vi "readRestek.vi"(10 "Port Name":refnum<visa-resource-name>) -> (2 "lpm":dbl)   [LabVIEW 2020]
panel:
  out "element":string
  out "string array":string[](array[string])
  out "Read":string="This is simulation mode"
  # "Reads data stream from Restek ProFLOW 6000 volumetric flowmeter"
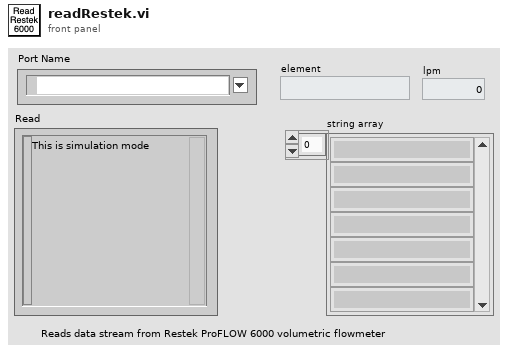
[diagram p1: front panel]
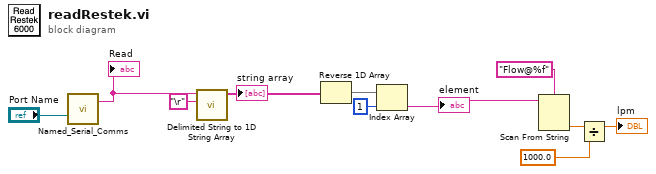
[diagram p0: block diagram]
diagram:
  n1 = call "Named_Serial_Comms.vi"("Port Name"="Port Name") -> ("Read"=w10:string)  [unwired: 10 in, 4 out]
  "Read" <- w10
  n2 = call <vilib>:"Delimited String to 1D String Array.vi"("delimiter"="\r", "delimited string"=w10) -> ("string array"=w8:string[])  [unwired: 9 in]
  "string array" <- w8
  n3 = Reverse 1D Array(array=w8) -> (reversed array=w7:string[])
  n4 = Index Array(array=w7, index=1) -> (element=w5:string)
  "element" <- w5
  n5 = Scan From String(format string="Flow@%f", input string=w5) -> (output 1=w4:dbl)  [unwired: 3 in, 3 out]
  n6 = Divide(x=w4, y=1000.0) -> (x/y=→"lpm":dbl)
